vi "Calculate Hot Goal.vi"(10 "Camera Samples":bool[](array[boolean])) -> (0 "Confident Answer?":bool, 2 "Right Hot?":bool)   [LabVIEW 2013]
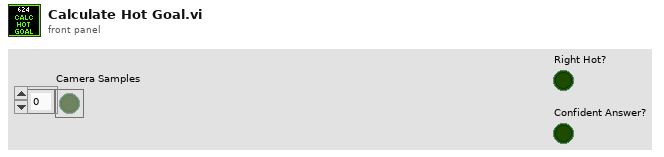
[diagram p1: front panel]
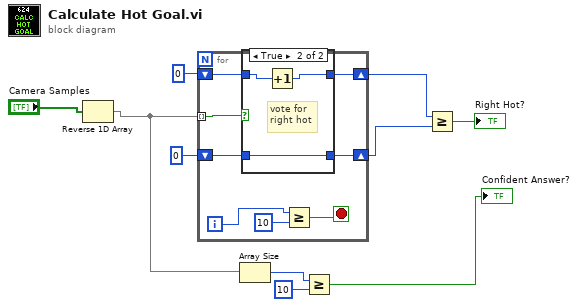
[diagram p0: block diagram]
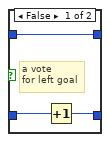
[diagram p2: hidden frame]
diagram:
  n1 = Reverse 1D Array(array="Camera Samples") -> (reversed array=w1:bool[])
  n2 = for {
    tunnel: w1 -> [w18] mode=indexing
    shift-right: [w16] -> w7
    shift-left: 0 -> [w17]
    shift-right: [w15] -> w6
    shift-left: 0 -> [w14]
    i -> [w12]
    stop <- w11 stop-if-true
    n3 = case shown="True" w18 {
      tunnel: w17 -> [w21 w24]
      tunnel: [w21 w23] -> w16
      tunnel: [w20 w22] -> w15
      tunnel: w14 -> [w19 w22]
      frame False {
        # "a vote \nfor left goal"
        n4 = Increment(x=w19) -> (x+1=w20:i32)
      }
      frame True {
        # "vote for\nright hot"
        n5 = Increment(x=w24) -> (x+1=w23:i32)
      }
    }
    n6 = Greater Or Equal?(x=w12, y=10) -> (x >= y?=w11:bool)
  }
  n7 = Array Size(array=w1) -> (size(s)=w5:i32)
  n8 = Greater Or Equal?(x=w5, y=10) -> (x >= y?=→"Confident Answer?":bool)
  n9 = Greater Or Equal?(x=w7, y=w6) -> (x >= y?=→"Right Hot?":bool)
